vi "OL_control.vi"(11 "goal_Tensions":dbl[](array[numeric])) -> (3 "can_Current":dbl[](array[numeric]))   [LabVIEW 2024]
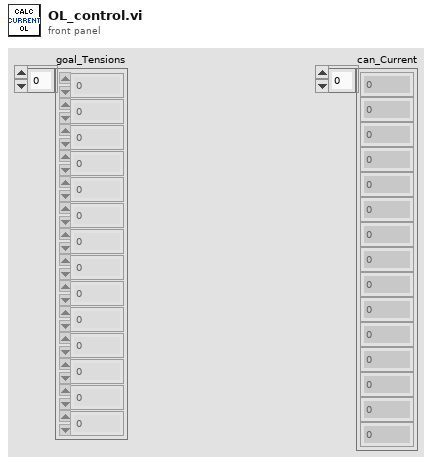
[diagram p1: front panel]
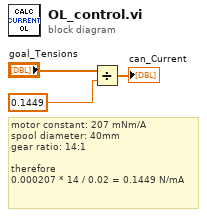
[diagram p0: block diagram]
diagram:
  # "motor constant: 207 mNm/A\nspool diameter: 40mm\ngear ratio: 14:1\n\ntherefore\n0.000207 * 14 / 0.02 = 0.1449 N/mA"
  n1 = Divide(x="goal_Tensions", y=0.1449) -> (x/y=→"can_Current":dbl[])
